vi "center2rectangle.vi"(1 "Center Y":sgl, 2 "Center X":sgl, 3 "Box Half Size":i32) -> (0 "Box Rectangle":T1)   [LabVIEW 2019]
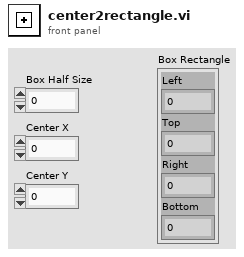
[diagram p1: front panel]
types:
  T1 = cluster{"Left":i32, "Top":i32, "Right":i32, "Bottom":i32}
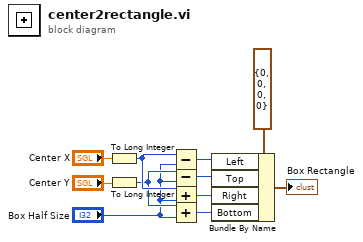
[diagram p0: block diagram]
diagram:
  n1 = To Long Integer(number="Center X") -> (32bit integer=w7:i32)
  n2 = To Long Integer(number="Center Y") -> (32bit integer=w6:i32)
  n3 = Subtract(x=w7, y="Box Half Size") -> (x-y=w9:i32)
  n4 = Subtract(x=w6, y="Box Half Size") -> (x-y=w8:i32)
  n5 = Add(x=w7, y="Box Half Size") -> (x+y=w11:i32)
  n6 = Add(x=w6, y="Box Half Size") -> (x+y=w10:i32)
  n7 = Bundle By Name(cluster=T1 {"Left"=0, "Top"=0, "Right"=0, "Bottom"=0} ("Rectangle"), "Left"=w9, "Top"=w8, "Right"=w11, "Bottom"=w10) -> (→"Box Rectangle":T1)
